vi "Test Execute SQL Query (string).vi"(8 "error in (no error)":errorcluster, 10 "query":string="SELECT * from employees;\nSELECT * from albums;\nSELECT 1+2;\nSELECT 3+4;", 11 "database in":path=path "C:/labview/sqlite_dbManager/test database/chinook.db") -> (0 "error out":errorcluster, 1 "Query Result":string[][](array[string]), 2 "nonzero result?":bool)   [LabVIEW 2020, in "sqlite3.lvlib"]
uses:
  sqlite3.lvlib
  sqlite/VIs/open v2.vi
  sqlite/VIs/prepare v2.vi
  sqlite/VIs/step.vi
  sqlite/VIs/column count.vi
  compound/Column.vi
  compound/Resolve Result Type.vi
  sqlite/VIs/finalize.vi
  sqlite/VIs/close v2.vi
  sqlite/subvi/Error Converter (ErrCode or Status).vi
  sqlite/VIs/column text.vi
  sqlite/VIs/column bytes.vi
  sqlite/VIs/column blob.vi
  utilities/MoveBlock.vi
  sqlite/VIs/column type.vi
  sqlite/VIs/errstr.vi
panel:
  in  "desired return type":string
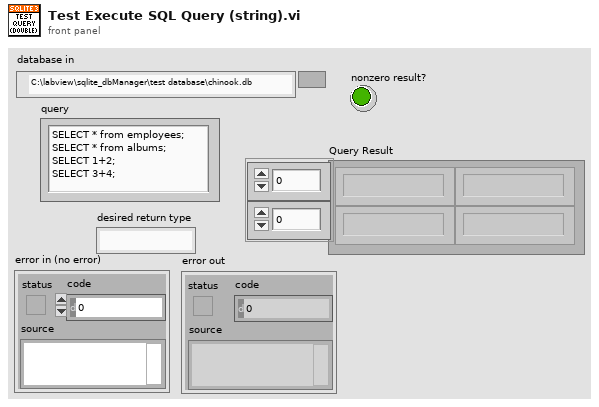
[diagram p1: front panel]
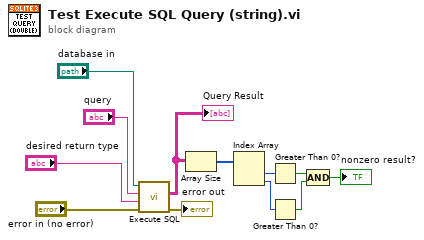
[diagram p0: block diagram]
diagram:
  n1 = call "Execute SQL.vi"("error in (no error)"="error in (no error)", "[disabled] return type (string)"="desired return type", "sql (string)"="query", "database in"="database in") -> ("error out"=→"error out":errorcluster, "Query Result"=w7:string[][])  [unwired: 6 in]
  "Query Result" <- w7
  n2 = Array Size(array=w7) -> (size(s)=w6:i32[])
  n3 = Index Array(array=w6) -> (element #1=w5:i32, element #2=w4:i32)  [unwired: 2 in]
  n4 = Greater Than 0?(x=w5) -> (x > 0?=w3:bool)
  n5 = Greater Than 0?(x=w4) -> (x > 0?=w2:bool)
  n6 = Compound Arithmetic op=AND(w3, w2) -> (→"nonzero result?":bool)
